vi "Build Channel Cluster Array.vi"() -> (3 "Channels":cluster{"Channels":T1[]})   [LabVIEW 2023, in "ChillerNew.lvclass"]
uses:
  ChillerNew.lvclass
  Utilities/Channel.ctl
  ChillerNew.lvclass/ChillerNew.ctl
  Utilities/Utilities.lvlib
panel:
  in  "Channels 2":cluster{"Channels":T1[]}
  in  "ChillerNew.lvclass":refnum<class "ChillerNew.lvclass">
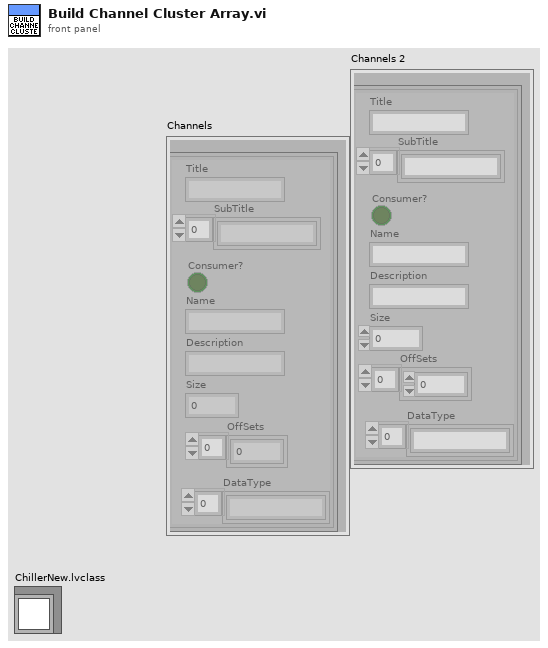
[diagram p1: front panel]
types:
  T1 = typedef "Utilities.lvlib/Channel.ctl" = cluster{"Title":string, "SubTitle":string[], "Consumer?":bool, "Name":string, "Description":string, "Size":i32, "OffSets":i32[], "DataType":string[]}
  T2 = cluster{"OnOffCtl":bool, "SP1":dbl, "Watchdog":i32}
  T3 = cluster{"OnOffSts":bool, "AV1":dbl, "WatchdogSTS":i32}
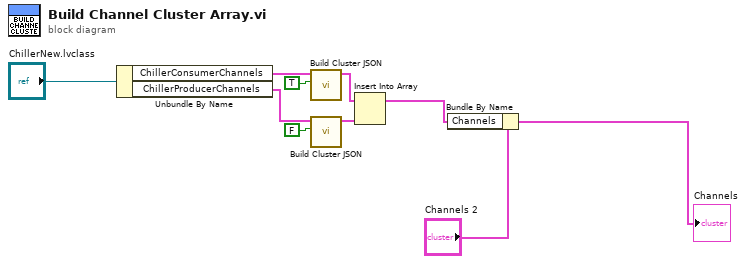
[diagram p0: block diagram]
diagram:
  n1 = Unbundle By Name("ChillerNew.lvclass") -> ("ChillerConsumerChannels"=w9:T2, "ChillerProducerChannels"=w8:T3)
  n2 = call "Build Cluster JSON.vi"("Consumer?"=TRUE, "Cluster"=w9) -> ("Array"=w5:T1[])  [unwired: 9 in]
  n3 = call "Build Cluster JSON.vi"("Consumer?"=FALSE, "Cluster"=w8) -> ("Array"=w4:T1[])  [unwired: 9 in]
  n4 = Insert Into Array(array=w5, new element=w4) -> (w2:T1[])  [unwired: 1 in]
  n5 = Bundle By Name(cluster="Channels 2", "Channels"=w2) -> (→"Channels":cluster{"Channels":T1[]})
